vi "Mutate FPGA Addon in SysDef.vi"(8 "error in (no error)":errorcluster, 11 "System Definition path in":path) -> (0 "error out":errorcluster, 3 "System Definition path out":path)   [LabVIEW 2018, in "FPGA Addon Test Class.lvclass"]
doc: "This utility VI applies mutation code to all of the FPGA Addon custom devices found in the target system definition file."
uses:
  FPGA Addon Test Class.lvclass
  NationalInstruments.VeriStand.SystemDefinitionAPI
  APIs/Scripting API/Scripting API.lvlib
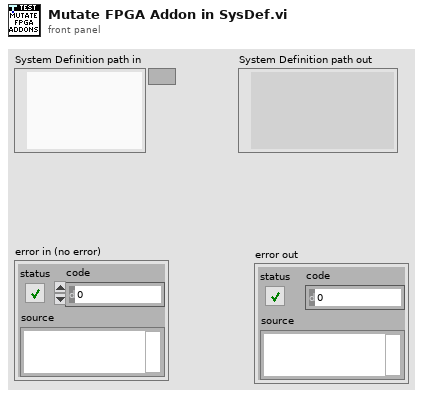
[diagram p1: front panel]
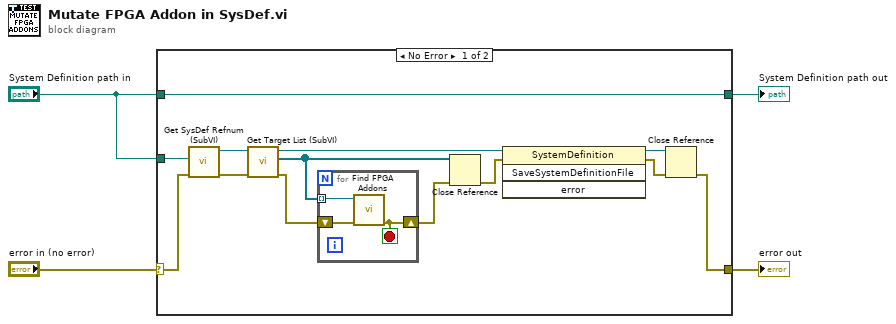
[diagram p0: block diagram]
diagram:
  n1 = case shown="No Error" "error in (no error)" {
    selector: "error in (no error)" -> [w6 w22]
    tunnel: "System Definition path in" -> [w8 _]
    tunnel: [w7 w22] -> w4
    tunnel: "System Definition path in" -> [w5 w21]
    tunnel: [w5 w21] -> w1
    frame No Error {
      n2 = call "Get SysDef Refnum (SubVI).vi"("error in (no error)"=w6, "System Definition path"=w8) -> ("error out"=w16:errorcluster, "SysDef Refnum out"=w17:refnum<k24>)  [unwired: 8 in]
      n3 = call "Get Target List (SubVI).vi"("error in (no error)"=w16, "SysDef Refnum in"=w17) -> ("error out"=w12:errorcluster, "Target List Refnums"=w11:refnum<k24>[], "SysDef Refnum out"=w15:refnum<k24>)  [unwired: 7 in]
      n4 = for {
        tunnel: w11 -> [w20] mode=indexing
        shift-right: [w18] -> w10
        shift-left: w12 -> [w19]
        stop <- w18 stop-if-true
        n5 = call "Find FPGA Addons.vi"("error in"=w19, "target in"=w20) -> ("error out"=w18:errorcluster)  [unwired: 6 in, 3 out]
      }
      n6 = Close Reference(reference=w11, error in (no error)=w10) -> (error out=w9:errorcluster)
      n7 = invoke class="SystemDefinition" method="SaveSystemDefinitionFile"(reference=w15, error in=w9) -> (reference out=w13:refnum<k24>, error out=w14:errorcluster)  [unwired: 2 in, 2 out]
      n8 = Close Reference(reference=w13, error in (no error)=w14) -> (error out=w7:errorcluster)
    }
    frame Error {
    }
  }
  "error out" <- w4
  "System Definition path out" <- w1
